vi "UpdateFilter.vi"(7 "LVWS Req":refnum<class "Web Request.lvclass">, 11 "State":u8) -> ()   [LabVIEW 2014]
uses:
  <vilib>/wsapi/Web Request.lvclass
  Controller/Messages/Change Filter State/Change Filter State.lvclass
  Controller/Messages/Update Switch State MSG/Update Switch MSG.lvclass/Update Switch MSG.ctl
  Controller/Messages/Update Switch State MSG/Write Val.vi
  Controller/Controller.lvclass
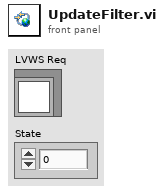
[diagram p1: front panel]
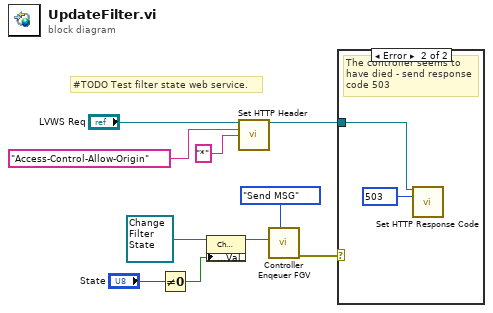
[diagram p0: block diagram]
diagram:
  # "#TODO Test filter state web service."
  n1 = Not Equal To 0?(x="State") -> (x != 0?=w4:bool)
  n2 = property class="Change Filter State MSG"(reference=refnum<class "Change Filter State.lvclass"> refnum ("Controller.lvlib:Change Filter State.lvclass"), "Accessors:Val"=w4) -> (reference out=w3:refnum<class "Change Filter State.lvclass">)  [unwired: 1 in, 1 out]
  n3 = call <vilib>:"Set HTTP Header.vi"("LabVIEW Web Service Request"="LVWS Req", "header"="Access-Control-Allow-Origin", "header value"="*") -> ("LabVIEW Web Service Request out"=w8:refnum<class "Web Request.lvclass">)  [unwired: 11 in, 1 out]
  n4 = call "Controller Enqeuer FGV.vi"("State"=enum16{"Store", "Send MSG"}."Send MSG", "MSG"=w3) -> ("error out"=w7:errorcluster)  [unwired: 9 in]
  n5 = case shown="Error" w7 {
    tunnel: w8 -> [_ w11]
    frame No Error {
    }
    frame Error {
      w12 = 503 items=["100"=100, "101"=101, "200"=200, "201"=201, "202"=202, "203"=203, "204"=204, "205"=205, "206"=206, "300"=300, "301"=301, "302"=302, "303"=303, "304"=304, "305"=305, "306"=306, "307"=307, "400"=400, "401"=401, "402"=402, "403"=403, "404"=404, "405"=405, "406"=406, "407"=407, "408"=408, "409"=409, "410"=410, "411"=411, "412"=412, "413"=413, "414"=414, "415"=415, "416"=416, "417"=417, "500"=500, "501"=501, "502"=502, "503"=503, "504"=504, "505"=505] ("response code (200)")
      # "The controller seems to have died - send response code 503"
      n6 = call <vilib>:"Set HTTP Response Code.vi"("LabVIEW Web Service Request"=w11, "response code (200)"=w12) -> ()  [unwired: 12 in, 2 out]
    }
  }
